vi "WifiConcat.vi"(1 "TUID":string="34002001180314080000000014541533") -> (0 "WIFIName":string)   [LabVIEW 2013]
panel:
  out "error out":errorcluster caption="错误输出"
  in  "error in":errorcluster caption="错误输入（无错误）"
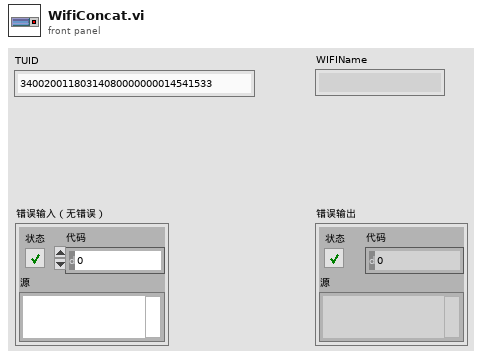
[diagram p1: front panel]
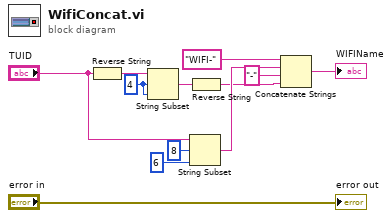
[diagram p0: block diagram]
diagram:
  w11 = 4 ("偏移量(0)")
  n1 = Reverse String(1:"TUID") -> (0:w12:string)
  n2 = String Subset(string=w12, offset (0)=w11, length (rest)=w11) -> (substring=w10:string)
  n3 = String Subset(string="TUID", offset (0)=8 ("偏移量(0)"), length (rest)=6 ("偏移量(0)")) -> (substring=w8:string)
  n4 = Reverse String(1:w10) -> (0:w5:string)
  n5 = Concatenate Strings("WIFI-", w8, "-", w5) -> (→"WIFIName":string)
  "error out" <- "error in"
